vi "SVT THD and Harmonic Components (Time) (1 Ch).vi"(0 "scaled signal [EU]":waveform(dbl), 2 "maximum harmonic":i32=-1, 3 "harmonics to visualize":i32[](array[numeric])=[-1], 5 "error in (no error)":errorcluster, 6 "desired units":T2, 9 "expected fundamental frequency [Hz]":dbl=-1.0 format="%.2f") -> (10 "actual maximum harmonic":i32=5, 11 "detected fundamental\nfrequency [Hz]":dbl format="%.2f", 12 "unit labels":T1, 13 "detected fundamental\namplitude":dbl format="%.2f", 14 "complex spectrum":T9={"complex spectrum response"={"f0"=0.0, "df"=1.0, "complex spectrum"=[]}, "spectrum info"={"channel name"="", "description"="", "x-axis units"=0, "spectral info"={"spectrum type"=enum."Power [Magnitude^2]", "linear/dB"=enum."linear", "window"=0, "window size"=0, "FFT size"=0}, "engineering units"=0, "custom label"="", "dB reference [EU]"=0.0, "peak units"=enum."rms", "weighting filter"=0, "spectral density?"=FALSE, "unit label"="", "spectrum skewed?"=FALSE, "complimentary spectrum units"=enum."none"}} {"spectrum info"."x-axis units" items=["Time (s)"=0, "Frequency-CB (Hz)"=1, "Frequency-CPB (Hz)"=1248, "Frequency-Arbitrary (Hz)"=2357, "Quefrency (s)"=2, "Revolutions (rev)"=3, "Order"=4, "Speed (RPM)"=11, "Speed (rad/s)"=21, "Index"=65535]; "spectrum info"."weighting filter" items=["Linear", "A-weighting", "B-weighting", "C-weighting", "ITU-R 468-4", "Dolby", "CCITT", "C-message", "Wb", "Wc", "Wd", "We", "Wf", "Wh", "Wj", "Wk", "Wm", "AES17 20 kHz lowpass", "AES17 40 kHz lowpass", "AES17 20 kHz highpass", "AES17 40 kHz highpass"]; "spectrum info"."dB reference [EU]" format="%.2f"; "spectrum info"."engineering units" items=["custom..."=0, "V"=1, "A"=21, "C"=30, "pC"=31, "s"=32, "-"=29, "Pa"=2, "N"=20, "g"=3, "m/s^2"=4, "m/s"=5, "m"=6, "mm/s"=12, "mm"=13, "micron/s"=14, "micron"=15, "in/s^2"=7, "in/s"=8, "in"=9, "mil/s"=10, "mil"=11, "rad/s^2"=16, "rad/s"=17, "rad"=18, "deg/s^2"=26, "deg/s"=27, "deg"=28, "RPM"=22, "cycle/s^2"=23, "Hz"=24, "cycle"=25, "strain"=19]; "spectrum info"."spectral info"."window" items=["None "=0, "Hanning"=1, "Hamming"=2, "Blackman-Harris"=3, "Exact Blackman"=4, "Blackman"=5, "Flat Top"=6, "4 Term B-Harris "=7, "7 Term B-Harris"=8, "Low Sidelobe"=9, "Force - Exponential"=10, "Gaussian"=62]; "complex spectrum response"."complex spectrum" format="%.2f"; "complex spectrum response"."df" format="%.2f"; "complex spectrum response"."f0" format="%.2f"}, 16 "THD":dbl format="%.2f", 17 "harmonic components":cluster{"frequency [Hz]":dbl, "amplitude":dbl}[](array[cluster]) {"amplitude" format="%.2f"; "frequency [Hz]" format="%.2f"}, 19 "error out":errorcluster)   [LabVIEW 2017, in "SoundVib_Distortion.lvlib"]
doc: "Performs a total harmonic distortion analysis, including measuring the fundamental tone and harmonics, and returns the detected fundamental frequency, detected fundamental amplitude, harmonic components, and total harmonic distortion (THD). Wire data to the <B>scaled signal [EU]</B> input to determine the polymorphic instance to use or manually select the instance.\n\nThe following formula calculates THD:\n\nTHD = H / F\n\nwhere H is the harmonic RMS level and F is the fundamental tone RMS level."
uses:
  <vilib>/addons/Sound and Vibration/svt_Distortion/SoundVib_Distortion.lvlib
  <vilib>/addons/_NISVFA/_Shared subVIs/Controls/svc_Spectrum Info.ctl
  <vilib>/addons/_NISVFA/_Shared subVIs/Controls/svc_X-Axis Units.ctl
  <vilib>/addons/_NISVFA/_Shared subVIs/Controls/svc_Spectrum Type.ctl
  <vilib>/addons/_NISVFA/_Shared subVIs/Controls/svc_Engineering Units Text Ring.ctl
  <vilib>/addons/_NISVFA/_Shared subVIs/Controls/svc_Weighting Filter Text Ring.ctl
  <vilib>/addons/_NISVFA/_Shared subVIs/Controls/svc_Complimentary Spectrum Units.ctl
  <vilib>/addons/_NISVFA/_Shared subVIs/Controls/svc_Window.ctl
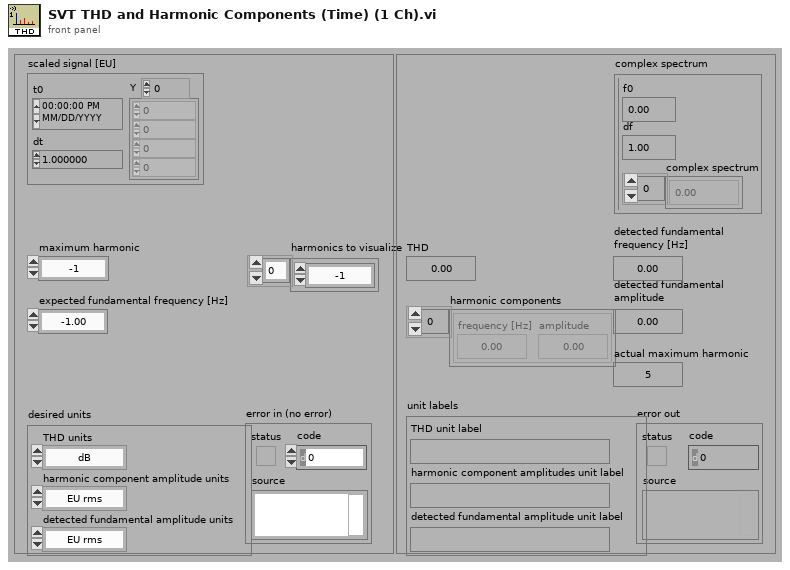
[diagram p1: front panel]
types:
  T1 = cluster{"THD unit label":string, "harmonic component amplitudes unit label":string, "detected fundamental amplitude unit label":string}
  T2 = cluster{"THD units":enum16{"dB", "linear ratio", "%"}, "harmonic component amplitude units":enum16{"EU rms", "EU peak", "EU peak-peak", "dB ref fund"}, "detected fundamental amplitude units":enum16{"EU rms", "EU peak", "EU peak-peak"}}
  T3 = typedef "svc_Spectrum Info.ctl" = cluster{"channel name":string, "description":string, "x-axis units":T4, "spectral info":cluster{"spectrum type":T5, "linear/dB":enum16{"linear", "dB"}, "window":u16, "window size":i32, "FFT size":i32}, "engineering units":T6, "custom label":string, "dB reference [EU]":dbl, "peak units":enum16{"rms", "peak", "peak-peak"}, "weighting filter":T7, "spectral density?":bool, "unit label":string, "spectrum skewed?":bool, "complimentary spectrum units":T8}
  T4 = typedef "svc_X-Axis Units.ctl" = u16
  T5 = typedef "svc_Spectrum Type.ctl" = enum16{"FFT Spectrum [complex]", "Amplitude [Magnitude]", "Power [Magnitude^2]", "Cross Spectrum [complex]", "Frequency Response [Complex]"}
  T6 = typedef "svc_Engineering Units Text Ring.ctl" = u16
  T7 = typedef "svc_Weighting Filter Text Ring.ctl" = u16
  T8 = typedef "svc_Complimentary Spectrum Units.ctl" = enum16{"none", "radians", "degrees", "cycles", "imaginary"}
  T9 = cluster{"complex spectrum response":cluster{"f0":dbl, "df":dbl, "complex spectrum":cdb[]}, "spectrum info":T3}
  T10 = cluster{"gain unit label":string, "phase unit label":string, "amplitude unit label":string}
  T11 = typedef "svc_Window.ctl" = u32
  T12 = cluster{"complex spectrum":cluster{"f0":dbl, "df":dbl, "complex spectrum":cdb[]}, "spectrum info":T3}
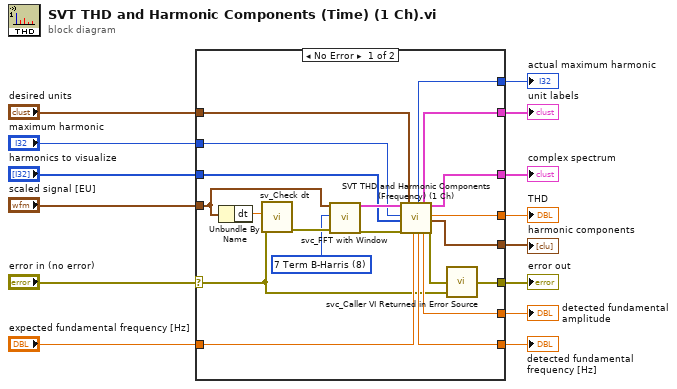
[diagram p0: block diagram]
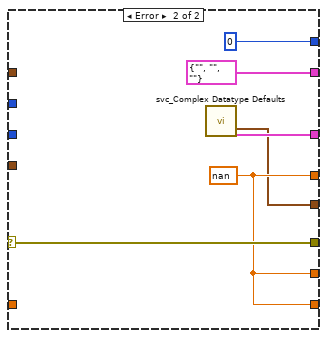
[diagram p2: hidden frame]
diagram:
  n1 = case shown="No Error" "error in (no error)" {
    selector: "error in (no error)" -> [w15 w40]
    tunnel: "scaled signal [EU]" -> [w17 _]
    tunnel: "expected fundamental frequency [Hz]" -> [w31 _]
    tunnel: [w24 w40] -> w12
    tunnel: [w33 w35] -> w9
    tunnel: [w22 w39] -> w10
    tunnel: [w23 w36] -> w8
    tunnel: [w30 w39] -> w7
    tunnel: [w29 w39] -> w6
    tunnel: "desired units" -> [w27 _]
    tunnel: [w28 T10 {"gain unit label"="", "phase unit label"="", "amplitude unit label"=""} ("unit labels")] -> w4
    tunnel: "maximum harmonic" -> [w26 _]
    tunnel: "harmonics to visualize" -> [w21 _]
    tunnel: [w20 0 ("actual maximum harmonic")] -> w1
    frame No Error {
      w18 = T11 8 items=["None ", "Hanning", "Hamming", "Blackman-Harris", "Exact Blackman", "Blackman", "Flat Top", "4 Term B-Harris ", "7 Term B-Harris", "Low Sidelobe"] ("window")
      n2 = Unbundle By Name(w17) -> ("dt"=w16:dbl)
      n3 = call <vilib>:"sv_Check dt.vi"("error in"=w15, "dt"=w16) -> ("error out"=w19:errorcluster)  [unwired: 8 in, 1 out]
      n4 = call <vilib>:"svc_FFT with Window.vi"("time signal in [EU]"=w17, "window"=w18, "error in (no error)"=w19) -> ("complex spectrum"=w34:T9, "error out"=w32:errorcluster)  [unwired: 15 in]
      n5 = call <vilib>:"SVT THD and Harmonic Components (Frequency) (1 Ch).vi"("complex spectrum"=w34, "maximum harmonic"=w26, "harmonics to visualize"=w21, "error in (no error)"=w32, "desired units"=w27, "expected fundamental frequency [Hz]"=w31) -> ("actual maximum harmonic"=w20:i32, "detected fundamental\nfrequency [Hz]"=w29:dbl, "unit labels"=w28:T1, "detected fundamental\namplitude"=w30:dbl, "complex spectrum"=w23:T9, "THD"=w22:dbl, "harmonic components"=w33:cluster{"frequency [Hz]":dbl, "amplitude":dbl}[], "error out"=w25:errorcluster)  [unwired: 6 in]
      n6 = call <vilib>:"svc_Caller VI Returned in Error Source.vi"("warning input to caller"=w15, "error in (no error)"=w25) -> ("error out"=w24:errorcluster)  [unwired: 3 in]
    }
    frame Error {
      w39 = nan ("SINAD")
      n7 = call <vilib>:"svc_Complex Datatype Defaults.vi"() -> ("empty array of peaks"=w35:cluster{"frequency":dbl, "value":dbl}[], "complex spectrum"=w36:T12)  [unwired: 11 in, 7 out]
    }
  }
  "THD" <- w10
  "error out" <- w12
  "harmonic components" <- w9
  "complex spectrum" <- w8
  "detected fundamental\nfrequency [Hz]" <- w6
  "detected fundamental\namplitude" <- w7
  "unit labels" <- w4
  "actual maximum harmonic" <- w1
